vi "USB.Check Multiple Devices using PID and VID.vi"(8 "error in":errorcluster, 10 "PID":string="2500", 11 "VID":string="28DE") -> (0 "error out":errorcluster, 1 "Subkey":string, 2 "Path":string, 3 "Found":bool)   [LabVIEW 2018]
uses:
  <vilib>/registry/registry.llb/Registry SAM.ctl
  <vilib>/registry/registry.llb/Registry RtKey.ctl
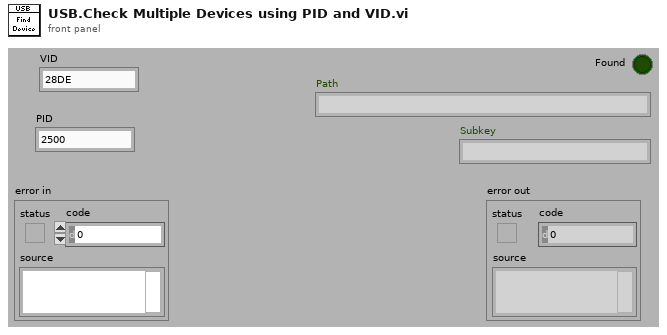
[diagram p1: front panel]
types:
  T1 = typedef "Registry RtKey.ctl" = enum32{"HKEY_CLASSES_ROOT", "HKEY_CURRENT_USER", "HKEY_LOCAL_MACHINE", "HKEY_USERS", "HKEY_PERFORMANCE_DATA", "HKEY_CURRENT_CONFIG", "HKEY_DYN_DATA"}
  T2 = typedef "Registry SAM.ctl" = enum32{"KEY_QUERY_VALUE", "KEY_SET_VALUE", "KEY_CREATE_SUB_KEY", "KEY_ENUMERATE_SUB_KEYS", "KEY_NOTIFY", "KEY_CREATE_LINK", "KEY_READ", "KEY_WRITE", "KEY_ALL_ACCESS", "KEY_READ | KEY_WRITE"}
  T3 = typedef "Registry refnum.ctl" = refnum<k1>
  T4 = cluster{"numValues":i32, "maxValueNameLen":i32, "maxValueDataLen":i32}
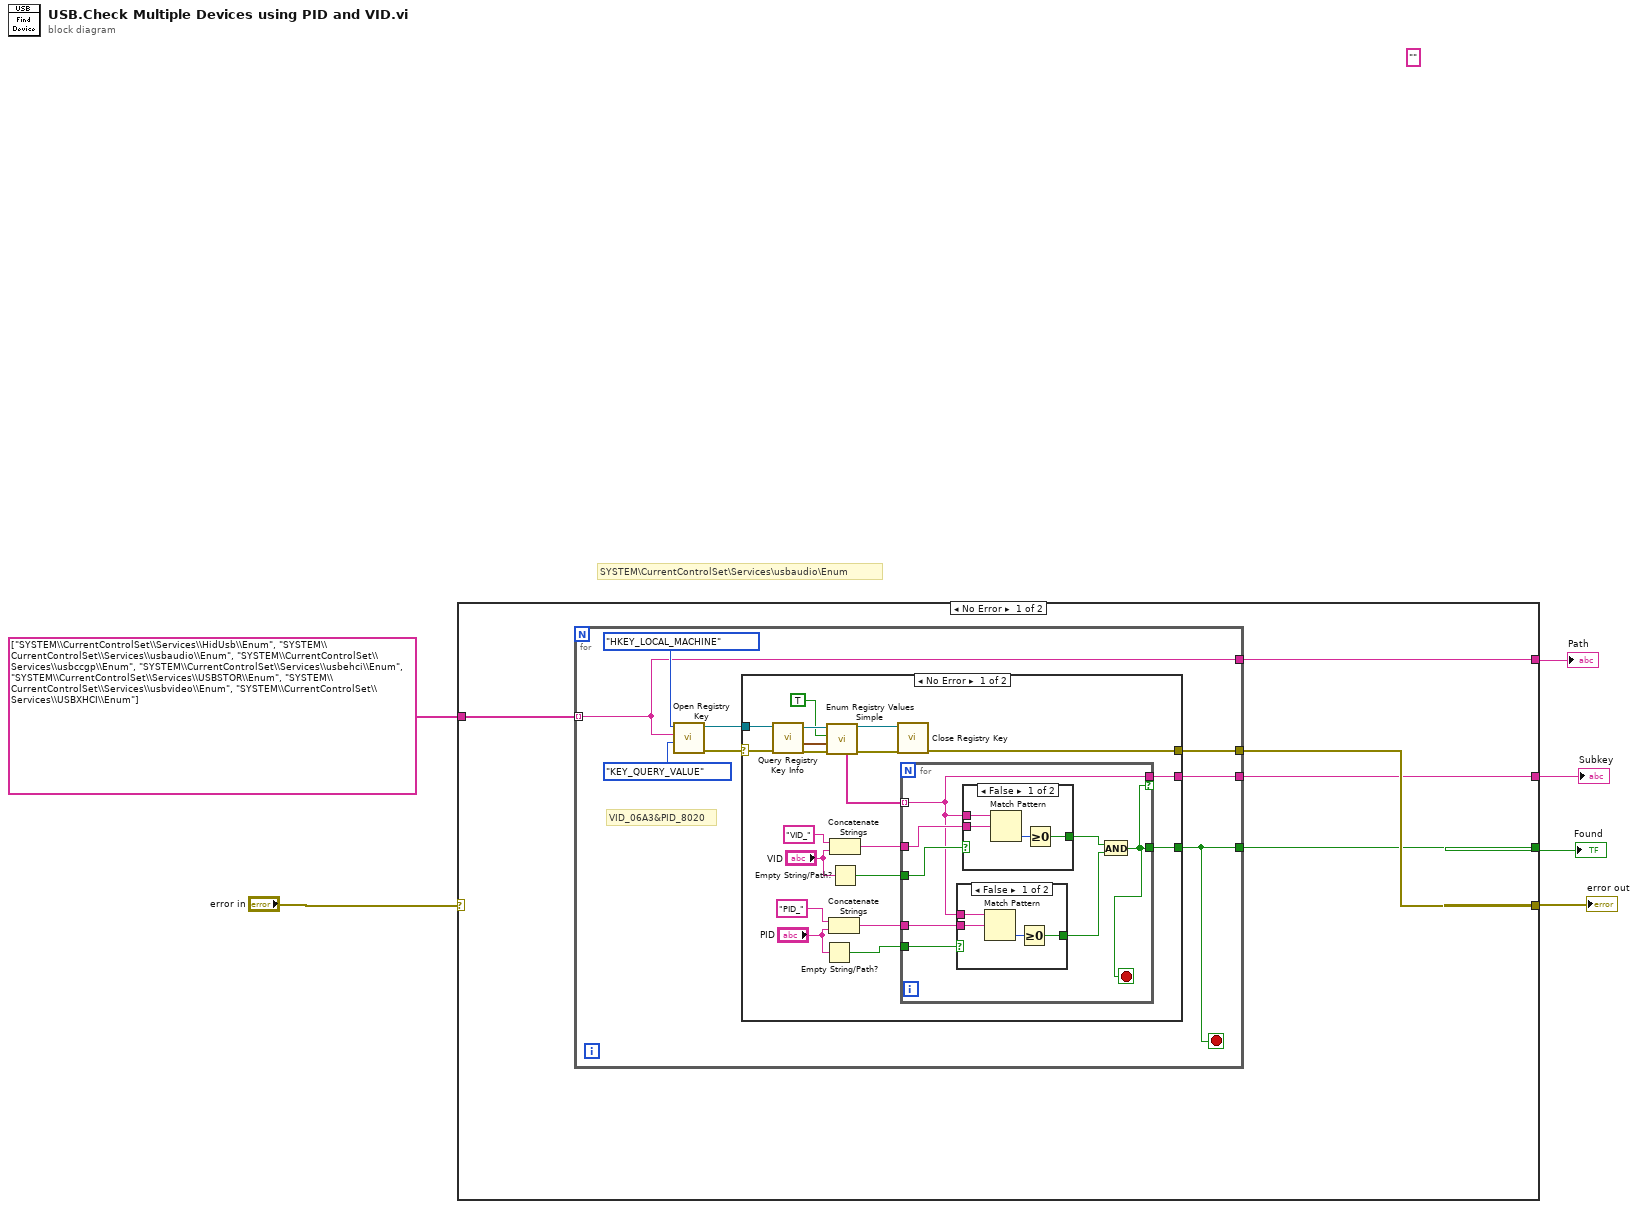
[diagram p0: block diagram]
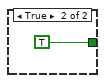
[diagram p2: hidden frame]
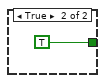
[diagram p3: hidden frame]
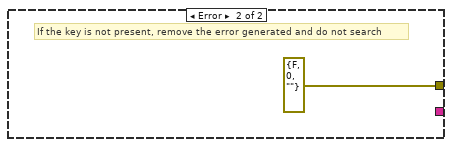
[diagram p4: hidden frame]
diagram:
  (unwired) ""
  # "SYSTEM\\CurrentControlSet\\Services\\usbaudio\\Enum"
  n1 = case shown="No Error" "error in" {
    selector: "error in" -> [_ w59]
    tunnel: [w11 w59] -> w6
    tunnel: [w10 _] -> w4
    tunnel: [w9 _] -> w3
    tunnel: string[] ["SYSTEM\\CurrentControlSet\\Services\\HidUsb\\Enum", "SYSTEM\\CurrentControlSet\\Services\\usbaudio\\Enum", "SYSTEM\\CurrentControlSet\\Services\\usbccgp\\Enum", "SYSTEM\\CurrentControlSet\\Services\\usbehci\\Enum", "SYSTEM\\CurrentControlSet\\Services\\USBSTOR\\Enum", "SYSTEM\\CurrentControlSet\\Services\\usbvideo\\Enum", "SYSTEM\\CurrentControlSet\\Services\\USBXHCI\\Enum"] -> [w8 _]
    tunnel: [w7 _] -> w1
    frame No Error {
      n2 = for {
        tunnel: [w16] -> w11
        tunnel: [w15] -> w10
        tunnel: [w14] -> w9
        tunnel: w8 -> [w12] mode=indexing
        tunnel: [w12] -> w7
        stop <- w14 stop-if-true
        # "VID_06A3&PID_8020"
        n3 = call <vilib>:"Open Registry Key.vi"("security access mask (KEY_READ | KEY_WRITE)"=Registry_SAM."KEY_QUERY_VALUE", "subkey"=w12, "root key (HKEY_LOCAL_MACHINE)"=Registry_RtKey."HKEY_LOCAL_MACHINE") -> ("error out"=w18:errorcluster, "refnum out"=w19:T3)  [unwired: 1 in, 6 out]
        n4 = case shown="No Error" w18 {
          selector: w18 -> [w38 _]
          tunnel: w19 -> [w39 _]
          tunnel: [w37 errorcluster {"status"=FALSE, "code"=0, "source"=""} ("error in (no error)")] -> w16
          tunnel: [w28 _] -> w14
          tunnel: [w27 _] -> w15
          frame No Error {
            n5 = call <vilib>:"Query Registry Key Info.vi"("error in (no error)"=w38, "refnum"=w39) -> ("error out"=w25:errorcluster, "value info"=w20:T4, "refnum out"=w26:T3)  [unwired: 7 out]
            n6 = Empty String/Path?(string/path="PID") -> (empty?=w32:bool)
            n7 = call <vilib>:"Enum Registry Values Simple.vi"("error in (no error)"=w25, "value info"=w20, "retrieve data? (F)"=TRUE, "refnum"=w26) -> ("error out"=w23:errorcluster, "refnum out"=w24:T3, "String/Binary data"=w21:string[])  [unwired: 2 in, 3 out]
            n8 = Concatenate Strings("PID_", "PID") -> (w34:string)
            n9 = Concatenate Strings("VID_", "VID") -> (w31:string)
            n10 = Empty String/Path?(string/path="VID") -> (empty?=w29:bool)
            n11 = call <vilib>:"Close Registry Key.vi"("error in (no error)"=w23, "refnum"=w24) -> ("error out"=w37:errorcluster)  [unwired: 5 out]
            n12 = for {
              tunnel: w21 -> [w43] mode=indexing
              tunnel: [w43] -> w27 if=w40
              tunnel: w31 -> [w45]
              tunnel: w34 -> [w47]
              tunnel: w32 -> [w46]
              tunnel: w29 -> [w44]
              tunnel: [w40] -> w28
              stop <- w40 stop-if-true
              n13 = case shown="False" w46 {
                tunnel: w47 -> [w55 _]
                tunnel: [w54 TRUE] -> w41
                tunnel: w43 -> [w53 _]
                frame False {
                  n14 = Match Pattern(string=w53, regular expression=w55) -> (offset past match=w56:i32)  [unwired: 1 in, 3 out]
                  n15 = Greater Or Equal To 0?(x=w56) -> (x >= 0?=w54:bool)
                }
                frame True {
                }
              }
              n16 = case shown="False" w44 {
                tunnel: w45 -> [w50 _]
                tunnel: [w49 TRUE] -> w42
                tunnel: w43 -> [w48 _]
                frame False {
                  n17 = Match Pattern(string=w48, regular expression=w50) -> (offset past match=w51:i32)  [unwired: 1 in, 3 out]
                  n18 = Greater Or Equal To 0?(x=w51) -> (x >= 0?=w49:bool)
                }
                frame True {
                }
              }
              n19 = And(x=w42, y=w41) -> (x .and. y?=w40:bool)
            }
          }
          frame Error {
            # "If the key is not present, remove the error generated and do not search"
          }
        }
      }
    }
    frame Error {
    }
  }
  "error out" <- w6
  "Found" <- w3
  "Subkey" <- w4
  "Path" <- w1
